vi "FindUnexpectedDepsOfLibraries.vi"(6 "Failures Indicator Ref":refnum<vi>, 8 "error in (no error)":errorcluster, 9 "Status Indicator Ref":refnum<vi>, 10 "Lvlib paths":path[](array[path]), 11 "CLI in":refnum<class "CLI.lvclass">) -> (0 "error out":errorcluster, 2 "Failures Array":T1[](array[typedef]), 3 "CLI out":refnum<class "CLI.lvclass">)   [LabVIEW 2023, in "CICD.lvlib"]
uses:
  CICD.lvlib
  Typedefs/DepsCheckResult.ctl
  <vilib>/Wiresmith Technology/G CLI/CLI Class/CLI.lvclass
  <vilib>/Utility/config.llb/NI_LVConfig.lvlib
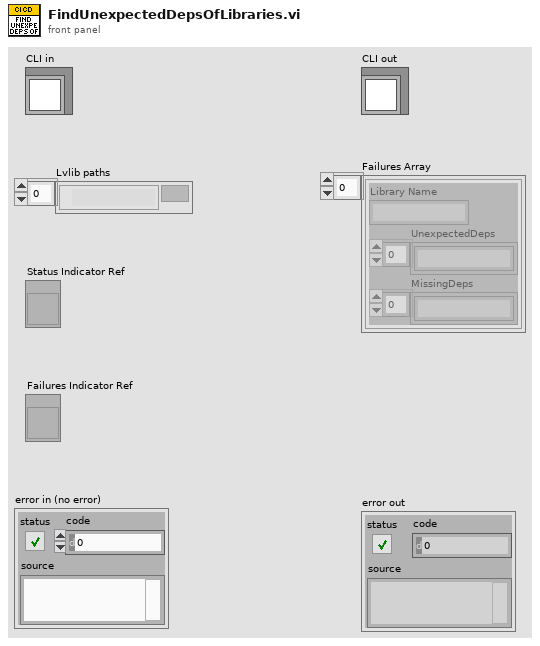
[diagram p1: front panel]
types:
  T1 = typedef "CICD.lvlib/DepsCheckResult.ctl" = cluster{"Library Name":string, "UnexpectedDeps":string[], "MissingDeps":string[]}
  T2 = typedef "NI_LVConfig.lvlib/Config Data RefNum.ctl" = refnum<k1>
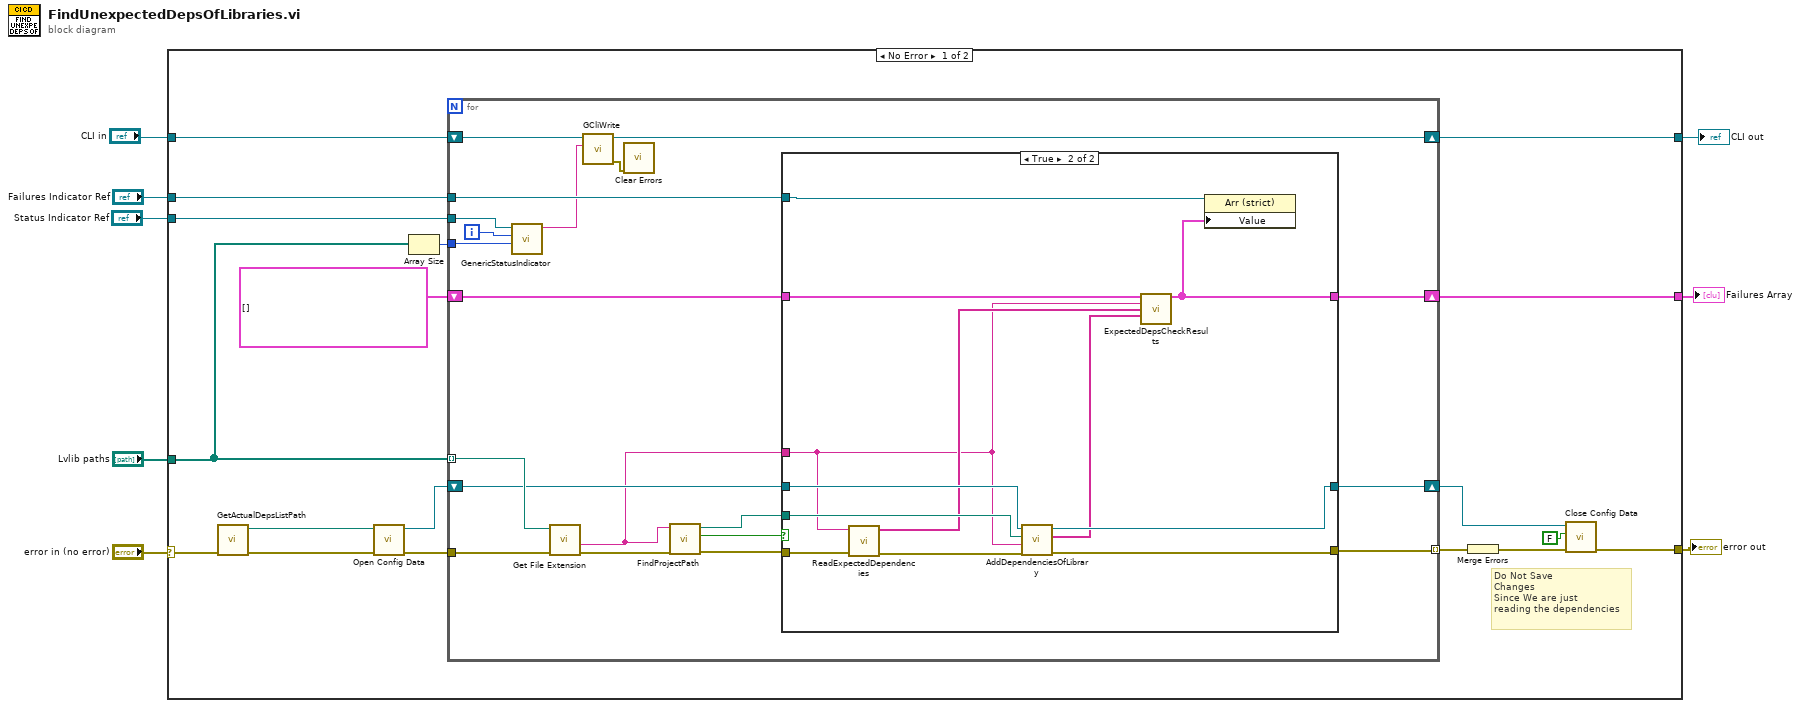
[diagram p0: block diagram]
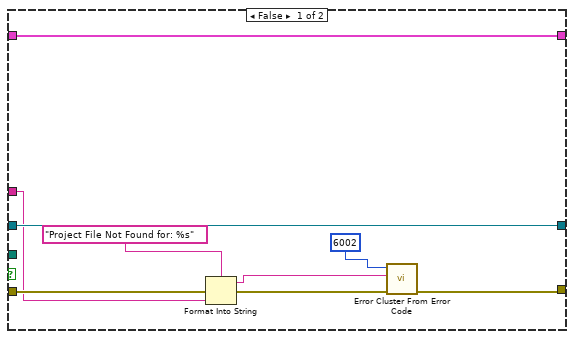
[diagram p2: hidden frame]
diagram:
  n1 = case shown="No Error" "error in (no error)" {
    selector: "error in (no error)" -> [w9 w69]
    tunnel: "Failures Indicator Ref" -> [w26 _]
    tunnel: "Status Indicator Ref" -> [w25 _]
    tunnel: [w24 _] -> w6
    tunnel: [w23 w68] -> w5
    tunnel: [w22 w69] -> w4
    tunnel: "CLI in" -> [w21 w68]
    tunnel: "Lvlib paths" -> [w15 _]
    frame No Error {
      # "Do Not Save\nChanges\nSince We are just\nreading the dependencies"
      n2 = call "GetActualDepsListPath.vi"("error in (no error)"=w9) -> ("error out"=w20:errorcluster, "ActualDepsListPath"=w19:path)  [unwired: 9 in]
      n3 = call <vilib>:"Open Config Data.vi"("error in (no error)"=w20, "configuration file path"=w19) -> ("error out"=w10:errorcluster, "refnum"=w12:T2)  [unwired: 7 in, 1 out]
      n4 = Array Size(array=w15) -> (size(s)=w16:i32)
      n5 = for {
        tunnel: w10 -> [w46]
        tunnel: w15 -> [w45] mode=indexing
        tunnel: [w29] -> w11 mode=indexing
        shift-right: [w39] -> w14
        shift-left: w12 -> [w40]
        tunnel: w16 -> [w38]
        shift-right: [w35] -> w24
        shift-left: T1[] [] -> [w36]
        shift-right: [w34] -> w23
        shift-left: w21 -> [w31]
        tunnel: w25 -> [w33]
        tunnel: w26 -> [w32]
        i -> [w37]
        n6 = call "GenericStatusIndicator.vi"("Total"=w38, "Current Iteration"=w37, "Status Indicator Ref In"=w33) -> ("CLI Status to Print"=w30:string)  [unwired: 8 in]
        n7 = call <vilib>:"Get File Extension.vi"("error in (no error)"=w46, "file"=w45) -> ("error out"=w44:errorcluster, "filename without extension"=w27:string)  [unwired: 5 in, 3 out]
        n8 = call "GCliWrite.vi"("Text to Write"=w30, "CLI in"=w31) -> ("error out"=w28:errorcluster, "CLI out"=w34:refnum<class "CLI.lvclass">)  [unwired: 8 in]
        n9 = call <vilib>:"Clear Errors.vi"("error in (no error)"=w28) -> ()  [unwired: 5 in, 2 out]
        n10 = call "FindProjectPath.vi"("error in (no error)"=w44, "Library Name"=w27) -> ("error out"=w42:errorcluster, "Found?"=w43:bool, "Project Path"=w41:path)  [unwired: 7 in]
        n11 = case shown="True" w43 {
          tunnel: w42 -> [w51 w64]
          tunnel: [w53 w62] -> w29
          tunnel: w41 -> [_ w67]
          tunnel: w40 -> [w55 w66]
          tunnel: [w55 w65] -> w39
          tunnel: w27 -> [w49 w56]
          tunnel: w36 -> [w54 w61]
          tunnel: [w54 w58] -> w35
          tunnel: w32 -> [_ w57]
          frame False {
            n12 = Format Into String(format string="Project File Not Found for: %s", error in=w51, w49) -> (resulting string=w48:string, error out=w47:errorcluster)  [unwired: 1 in]
            n13 = call <vilib>:"Error Cluster From Error Code.vi"("error in (no error)"=w47, "error message (\"\")"=w48, "error code (0)"=6002) -> ("error out"=w53:errorcluster)  [unwired: 6 in]
          }
          frame True {
            n14 = call "ReadExpectedDependencies.vi"("error in (no error)"=w64, "Library Name"=w56) -> ("error out"=w63:errorcluster, "ExpectedDependencies"=w60:string[])  [unwired: 6 in, 2 out]
            n15 = call "AddDependenciesOfLibrary.vi"("error in (no error)"=w63, "LibraryName"=w56, "Project Path"=w67, "Config Refnum in"=w66) -> ("error out"=w62:errorcluster, "ActualDependencies"=w59:string[], "Config Refnum out"=w65:T2)  [unwired: 5 in]
            n16 = call "ExpectedDepsCheckResults.vi"("ResultsArray"=w61, "Library Name"=w56, "ExpectedDependencies"=w60, "ActualDependencies"=w59) -> ("ResultsArray out"=w58:T1[])  [unwired: 11 in]
            n17 = property class="Arr (strict)"(reference=w57, "Value"=w58) -> ()  [unwired: 1 in, 2 out]
          }
        }
      }
      n18 = Merge Errors(w11) -> (w13:errorcluster)
      n19 = call <vilib>:"Close Config Data.vi"("error in (no error)"=w13, "write file if changed (T)"=FALSE, "refnum"=w14) -> ("error out"=w22:errorcluster)  [unwired: 7 in, 1 out]
    }
    frame Error {
    }
  }
  "Failures Array" <- w6
  "CLI out" <- w5
  "error out" <- w4
